vi "Replicate Action.vi"(10 "Square Type":refnum<class "Square.lvclass">, 11 "Direction":T1) -> (3 "Run Result":T2)   [LabVIEW 2020, in "SquareBattle.lvlib"]
doc: "Creates a replication action Run Result. The specified square type will be created in the specified direction. This can be a copy of this same class or it can be a different square type. Using different square classes can be a convenient way to encapsulate different behaviors within the same team of squares."
uses:
  SquareBattle.lvlib
  Run Result.ctl
  Square/Square.lvclass
  Action.ctl
  Direction.ctl
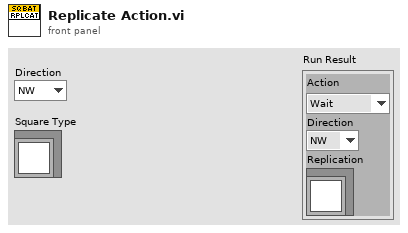
[diagram p1: front panel]
types:
  T1 = typedef "SquareBattle.lvlib/Direction.ctl" = enum16{"NW", "N", "NE", "E", "SE", "S", "SW", "W"}
  T2 = typedef "SquareBattle.lvlib/Run Result.ctl" = cluster{"Action":T3, "Direction":T1, "Replication":refnum<class "Square.lvclass">}
  T3 = typedef "SquareBattle.lvlib/Action.ctl" = enum16{"Wait", "Move", "Attack", "Replicate"}
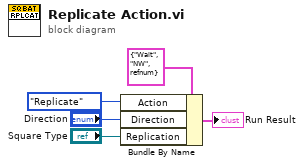
[diagram p0: block diagram]
diagram:
  n1 = Bundle By Name(cluster=T2 {"Action"=enum."Wait", "Direction"=enum."NW", "Replication"=refnum} ("Run Result"), "Action"=Action."Replicate", "Direction"="Direction", "Replication"="Square Type") -> (→"Run Result":T2)
